vi "accum-array-to-sizeN-and-pop.vi"(6 "Nsize":i32, 8 "new-data-in":dbl[][](array[numeric]), 11 "old-data-in":dbl[][](array[numeric])) -> (0 "popped-data":dbl[][](array[numeric]), 1 "new-data-ready":bool, 3 "old-data-out":dbl[][](array[numeric]))   [LabVIEW 2017]
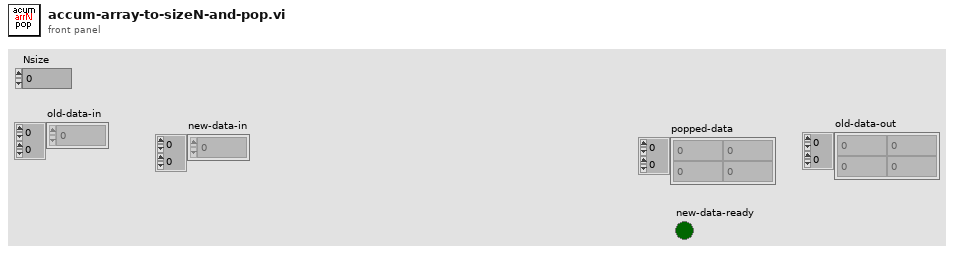
[diagram p1: front panel]
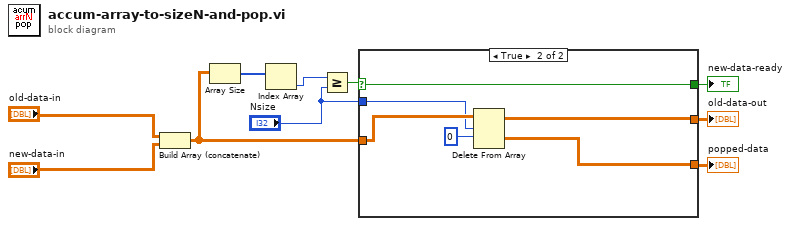
[diagram p0: block diagram]
diagram:
  n1 = Build Array (concatenate)("old-data-in", "new-data-in") -> (w10:dbl[][])
  n2 = Array Size(array=w10) -> (size(s)=w9:i32[])
  n3 = Index Array(array=w9) -> (element=w7:i32)  [unwired: 1 in]
  n4 = Greater Or Equal?(x=w7, y="Nsize") -> (x >= y?=w8:bool)
  n5 = case shown="True" w8 {
    selector: w8 -> [w11 w18]
    tunnel: [w12 w14] -> w2
    tunnel: w10 -> [w12 w17]
    tunnel: [w11 w18] -> w4
    tunnel: "Nsize" -> [_ w15]
    tunnel: [_ w13] -> w5
    frame False {
    }
    frame True {
      n6 = Delete From Array(array=w17, length=w15, index (row)=0 ("index")) -> (deleted portion=w13:dbl[][], array with subset deleted=w14:dbl[][])  [unwired: 1 in]
    }
  }
  "popped-data" <- w5
  "new-data-ready" <- w4
  "old-data-out" <- w2
